vi "CNR_CalcROIs.vi"(8 "Cut":i32, 9 "Background Size":i32, 10 "LOCH ROI Size":i32, 11 "Point":T1 {"Y" format="%.2f"; "X" format="%.2f"}) -> (0 "CutOff ROI":i32[](array[numeric]), 1 "Hole ROI":i32[](array[numeric]), 2 "Mask Insertion Point":i32[](array[numeric]), 3 "Background ROI":i32[](array[numeric]))   [LabVIEW 2023]
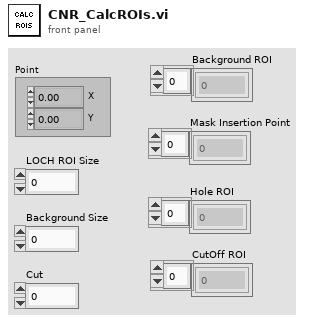
[diagram p1: front panel]
types:
  T1 = typedef "IMAQ Point" = cluster{"X":sgl, "Y":sgl}
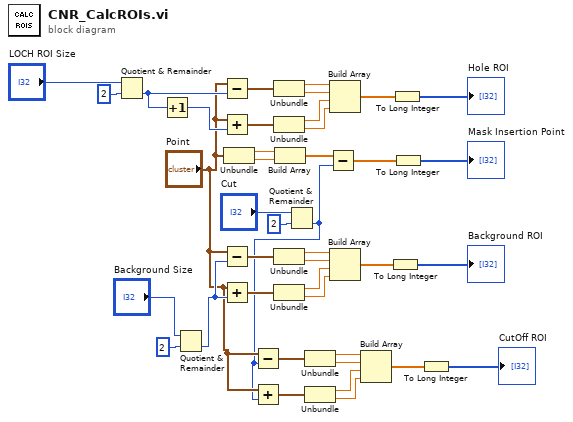
[diagram p0: block diagram]
diagram:
  n1 = Quotient & Remainder(x="LOCH ROI Size", y=2) -> (floor(x/y)=w40:i32)  [unwired: 1 out]
  n2 = Increment(x=w40) -> (x+1=w39:i32)
  n3 = Quotient & Remainder(x="Background Size", y=2) -> (floor(x/y)=w11:i32)  [unwired: 1 out]
  n4 = Subtract(x="Point", y=w40) -> (x-y=w19:T1)
  n5 = Add(x="Point", y=w39) -> (x+y=w20:T1)
  n6 = Subtract(x="Point", y=w11) -> (x-y=w28:T1)
  n7 = Add(x="Point", y=w11) -> (x+y=w29:T1)
  n8 = Unbundle("Point") -> ("X"=w32:sgl, "Y"=w33:sgl)
  n9 = Unbundle(w19) -> ("X"=w30:sgl, "Y"=w31:sgl)
  n10 = Unbundle(w20) -> ("X"=w21:sgl, "Y"=w22:sgl)
  n11 = Unbundle(w28) -> ("X"=w27:sgl, "Y"=w26:sgl)
  n12 = Unbundle(w29) -> ("X"=w25:sgl, "Y"=w24:sgl)
  n13 = Build Array(w32, w33) -> (w34:sgl[])
  n14 = Quotient & Remainder(x="Cut", y=2) -> (floor(x/y)=w1:i32)  [unwired: 1 out]
  n15 = Subtract(x="Point", y=w1) -> (x-y=w4:T1)
  n16 = Add(x="Point", y=w1) -> (x+y=w3:T1)
  n17 = Unbundle(w4) -> ("X"=w5:sgl, "Y"=w6:sgl)
  n18 = Unbundle(w3) -> ("X"=w7:sgl, "Y"=w8:sgl)
  n19 = Subtract(x=w34, y=w1) -> (x-y=w15:sgl[])
  n20 = Build Array(w30, w31, w21, w22) -> (w23:sgl[])
  n21 = Build Array(w27, w26, w25, w24) -> (w17:sgl[])
  n22 = Build Array(w5, w6, w7, w8) -> (w9:sgl[])
  n23 = To Long Integer(number=w17) -> (32bit integer=→"Background ROI":i32[])
  n24 = To Long Integer(number=w23) -> (32bit integer=→"Hole ROI":i32[])
  n25 = To Long Integer(number=w15) -> (32bit integer=→"Mask Insertion Point":i32[])
  n26 = To Long Integer(number=w9) -> (32bit integer=→"CutOff ROI":i32[])
